vi "Harry_kane_matlab_test.vi"() -> ()   [LabVIEW 2013]
uses:
  <vilib>/imath/engines/lvmath2/RunTimeEngine/ErrorHandling/NIMS_Finalize Error.vi
  <vilib>/imath/engines/lvmath2/RunTimeEngine/Managers/WorkSpace/UID Generator.vi
  <vilib>/imath/engines/lvmath2/RunTimeEngine/VariableToken/NIMS_VariableToken_CondDefined.vi
  <instcachedir>/0/NIMS_VariableToken_CondDefined_9DC5CEC47F8146B087FA2781C705B229.lvgen/NIMS_VariableToken_CondDefined_9DC5CEC47F8146B087FA2781C705B229_001.vi
  <vilib>/imath/engines/lvmath/Functions/Error Handling/MergeErrorsWrapper.vi
  <vilib>/imath/engines/lvmath2/RunTimeEngine/Managers/SymbolTable/Clear UID.vi
  <vilib>/imath/engines/lvmath2/RunTimeEngine/NodeEndStatement/NIMS_NodeEndStatement_Output.vi
  <instcachedir>/0/NIMS_NodeEndStatement_Output_53EC0D466D134D7ABD903AC30B43404B.lvgen/NIMS_NodeEndStatement_Output_53EC0D466D134D7ABD903AC30B43404B_011.vi
  <instcachedir>/0/NIMS_NodeEndStatement_Output_53EC0D466D134D7ABD903AC30B43404B.lvgen/NIMS_NodeEndStatement_Output_53EC0D466D134D7ABD903AC30B43404B_002.vi
  <vilib>/imath/engines/lvmath2/RunTimeEngine/RunTimeType/NIMS_RunTimeType_From StrictType (excl LVString).vi
  <instcachedir>/0/NIMS_RunTimeType_From StrictType (excl LVString)_4DEE718D6EB74582AA20236969C084FC.lvgen/NIMS_RunTimeType_From StrictType (excl LVString)_4DEE718D6EB74582AA20236969C084FC_000.vi
  <vilib>/imath/engines/lvmath2/RunTimeEngine/LocalVariableDefStatement/MC_LocalVariableDefStatement_Display.vi
  <vilib>/imath/engines/lvmath2/RunTimeEngine/IndexRead/NIMS V(S).vi
  <instcachedir>/0/NIMS V(S)_0488751826AF41519A22953C041130DC.lvgen/NIMS V(S)_0488751826AF41519A22953C041130DC_002.vi
  <vilib>/imath/engines/lvmath2/RunTimeEngine/BuiltInFunctions/max/2 inputs/NIMS_max(RG,RG)-no size check.vi
  <instcachedir>/0/NIMS_max(RG,RG)-no size check_F871939977644B7683C1350DCCAD7557.lvgen/NIMS_max(RG,RG)-no size check_F871939977644B7683C1350DCCAD7557_001.vi
  <vilib>/imath/engines/lvmath2/RunTimeEngine/ErrorHandling/NIMS_Create Error From Enums.vi
  <vilib>/imath/engines/lvmath2/RunTimeEngine/RangeToken/NIMS_Range_R2 - Integer.vi
  <instcachedir>/0/NIMS_Range_R2 - Integer_C51C130E5EA5464EA148B28CDAB9615A.lvgen/NIMS_Range_R2 - Integer_C51C130E5EA5464EA148B28CDAB9615A_000.vi
  <vilib>/imath/engines/lvmath2/RunTimeEngine/CommandStatement/MC_CommandStatement_break.vi
  <vilib>/imath/engines/lvmath2/RunTimeEngine/VariableToken/NIMS_VariableToken_CondDefinedDefinedByReplace.vi
  <instcachedir>/0/NIMS_VariableToken_CondDefinedDefinedByReplace_D162CFFC24174562A9FEA619A91E1A56.lvgen/NIMS_VariableToken_CondDefinedDefinedByReplace_D162CFFC24174562A9FEA619A91E1A56_002.vi
  <vilib>/imath/engines/lvmath2/RunTimeEngine/IndexRead/NIMS M(S).vi
  <instcachedir>/0/NIMS M(S)_B826C018497E4940AE96BD27B540B6FB.lvgen/NIMS M(S)_B826C018497E4940AE96BD27B540B6FB_000.vi
  <vilib>/imath/engines/lvmath2/RunTimeEngine/IndexReplace/NIMS V(S)=S.vi
  <instcachedir>/0/NIMS V(S)=S_66A18068148B4981A312229A93EA5C06.lvgen/NIMS V(S)=S_66A18068148B4981A312229A93EA5C06_000.vi
  <instcachedir>/0/NIMS V(S)_0488751826AF41519A22953C041130DC.lvgen/NIMS V(S)_0488751826AF41519A22953C041130DC_000.vi
  <vilib>/imath/engines/lvmath2/RunTimeEngine/BuiltInFunctions/min/2 inputs/NIMS_min(RG,RG)-no size check.vi
  <instcachedir>/0/NIMS_min(RG,RG)-no size check_7F67BAB91AFC452D9517D2EA1C8F5F88.lvgen/NIMS_min(RG,RG)-no size check_7F67BAB91AFC452D9517D2EA1C8F5F88_001.vi
  <vilib>/imathl/engines/lvmath/Functions/Error Handling/Create Error.vi
  <instcachedir>/0/NIMS_VariableToken_CondDefined_9DC5CEC47F8146B087FA2781C705B229.lvgen/NIMS_VariableToken_CondDefined_9DC5CEC47F8146B087FA2781C705B229_003.vi
  <vilib>/imath/engines/lvmath2/RunTimeEngine/BuiltInFunctions/length/NIMS_length(GV).vi
  <instcachedir>/0/NIMS_length(GV)_08A3D13377FD4E4B96F5795FBF3698FA.lvgen/NIMS_length(GV)_08A3D13377FD4E4B96F5795FBF3698FA_000.vi
  <instcachedir>/0/NIMS_VariableToken_CondDefinedDefinedByReplace_D162CFFC24174562A9FEA619A91E1A56.lvgen/NIMS_VariableToken_CondDefinedDefinedByReplace_D162CFFC24174562A9FEA619A91E1A56_001.vi
  <vilib>/imath/engines/lvmath2/RunTimeEngine/IndexReplace/NIMS M(S,S)=S.vi
  <instcachedir>/0/NIMS M(S,S)=S_EC2A86BD47664E68AE45685B0A86CA9E.lvgen/NIMS M(S,S)=S_EC2A86BD47664E68AE45685B0A86CA9E_000.vi
  <vilib>/imath/engines/lvmath2/RunTimeEngine/BuiltInFunctions/length/NIMS_length(GM).vi
  <instcachedir>/0/NIMS_length(GM)_47CEC356FCE0482D9BA47DC61C99F2C7.lvgen/NIMS_length(GM)_47CEC356FCE0482D9BA47DC61C99F2C7_000.vi
  <vilib>/imath/engines/lvmath2/RunTimeEngine/IndexRead/NIMS M(S,S).vi
  <instcachedir>/0/NIMS M(S,S)_AC51E74150A542F7991B9634C66F3096.lvgen/NIMS M(S,S)_AC51E74150A542F7991B9634C66F3096_000.vi
  <vilib>/vision/NI_Vision_Development_Module.lvlib
  <vilib>/imath/engines/lvmath2/RunTimeEngine/Managers/SymbolTable/NIMS_WorkSpace.lvlib
panel:
  in  "Tab Control":enum32{"DIP", "Histogram", "Raw Image"}(tab)
  out "Calibrated":T1(plugin-control)
  in  "Capture image":bool
  in  "Stop":bool
  in  "Calibrate":bool
  out "Puck Array From Reference (cm)":dbl[][](array[numeric])
  out "Player Array From Reference (cm)":dbl[][](array[numeric])
  out "Binary":T1(plugin-control)
  out "Rebound Shots":T1(plugin-control)
  out "Histogram":T2(graph)
  out "Image in":T1(plugin-control)
  out "Puck position pixels":dbl[][](array[numeric])
  out "Player Position Pixels":dbl[][](array[numeric])
  out "appended array":cluster{"X":sgl, "Y":sgl}[](array[cluster])
  out "R":i32
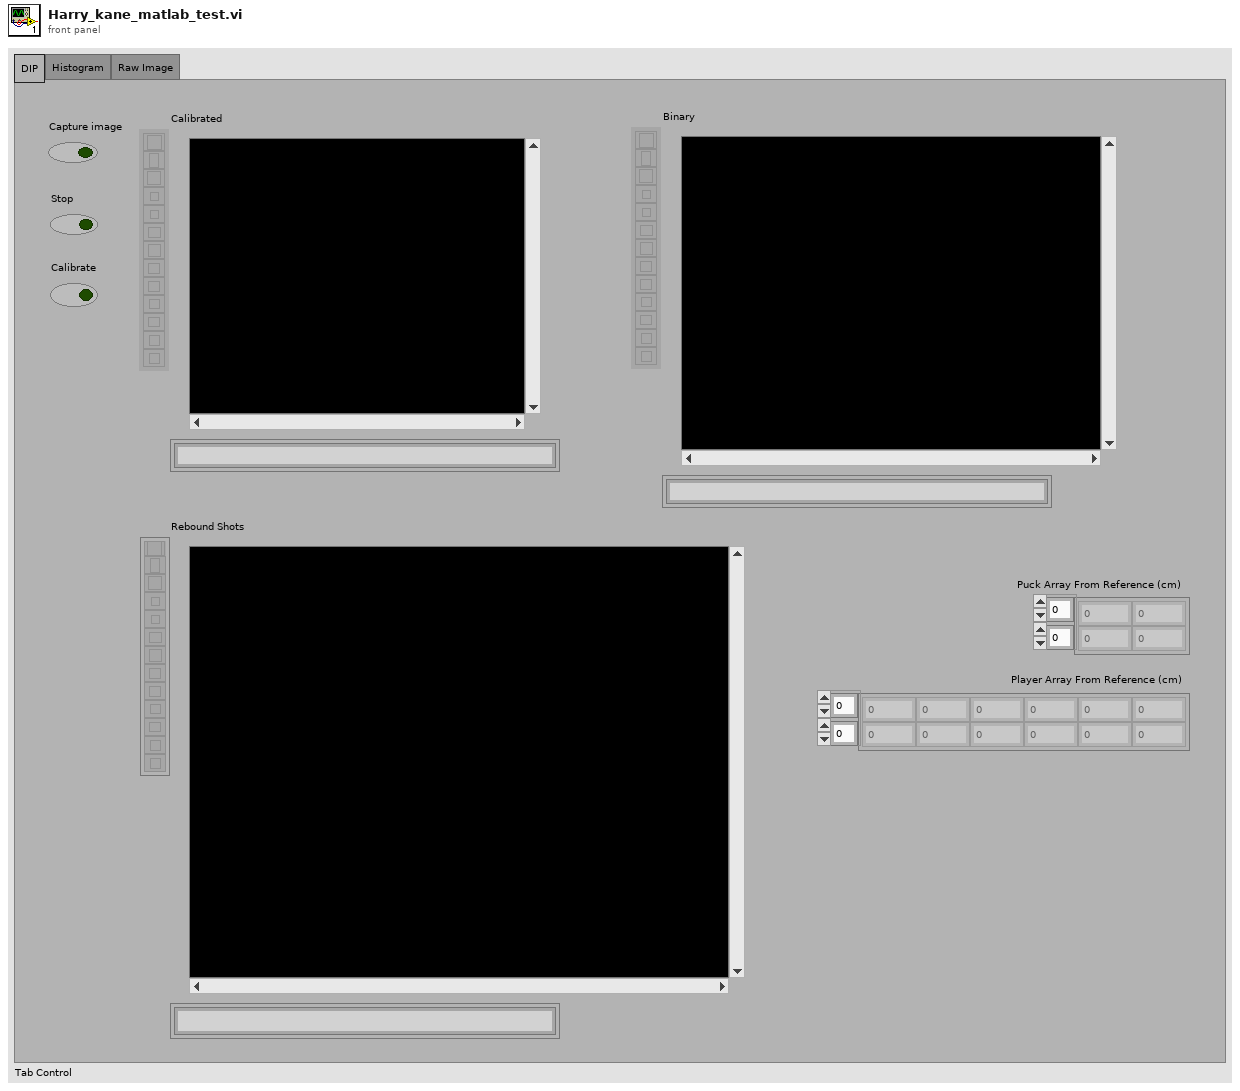
[diagram p1: front panel]
types:
  T1 = typedef "IMAQ Image.ctl" = refnum<image>
  T2 = cluster{"Starting Value":sgl, "Incremental Value":sgl, "Histogram":u32[]}
  T3 = typedef "Image Type" = u32
  T4 = cluster{"Point1 (Pixels)":cluster{"X":sgl, "Y":sgl}, "Point2 (Pixels)":cluster{"X":sgl, "Y":sgl}, "Point1 (Real-World)":cluster{"X":sgl, "Y":sgl}, "Point2 (Real-World)":cluster{"X":sgl, "Y":sgl}, "Angle (Pixel)":dbl, "Angle (Real-World)":dbl, "Score":dbl, "Straightness":dbl, "Average SNR (db)":dbl, "Calibration Valid":bool}
  T5 = cluster{"Start Point":cluster{"X":sgl, "Y":sgl}, "End Point":cluster{"X":sgl, "Y":sgl}, "Length":dbl, "Orientation":dbl, "Score":dbl}[]
  T6 = cluster{"Point1 (Pixels)":cluster{"X":sgl, "Y":sgl}, "Point2 (Pixels)":cluster{"X":sgl, "Y":sgl}}
  T7 = cluster{"Start Point":cluster{"X":sgl, "Y":sgl}, "End Point":cluster{"X":sgl, "Y":sgl}, "Length":dbl, "Orientation":dbl, "Score":dbl}
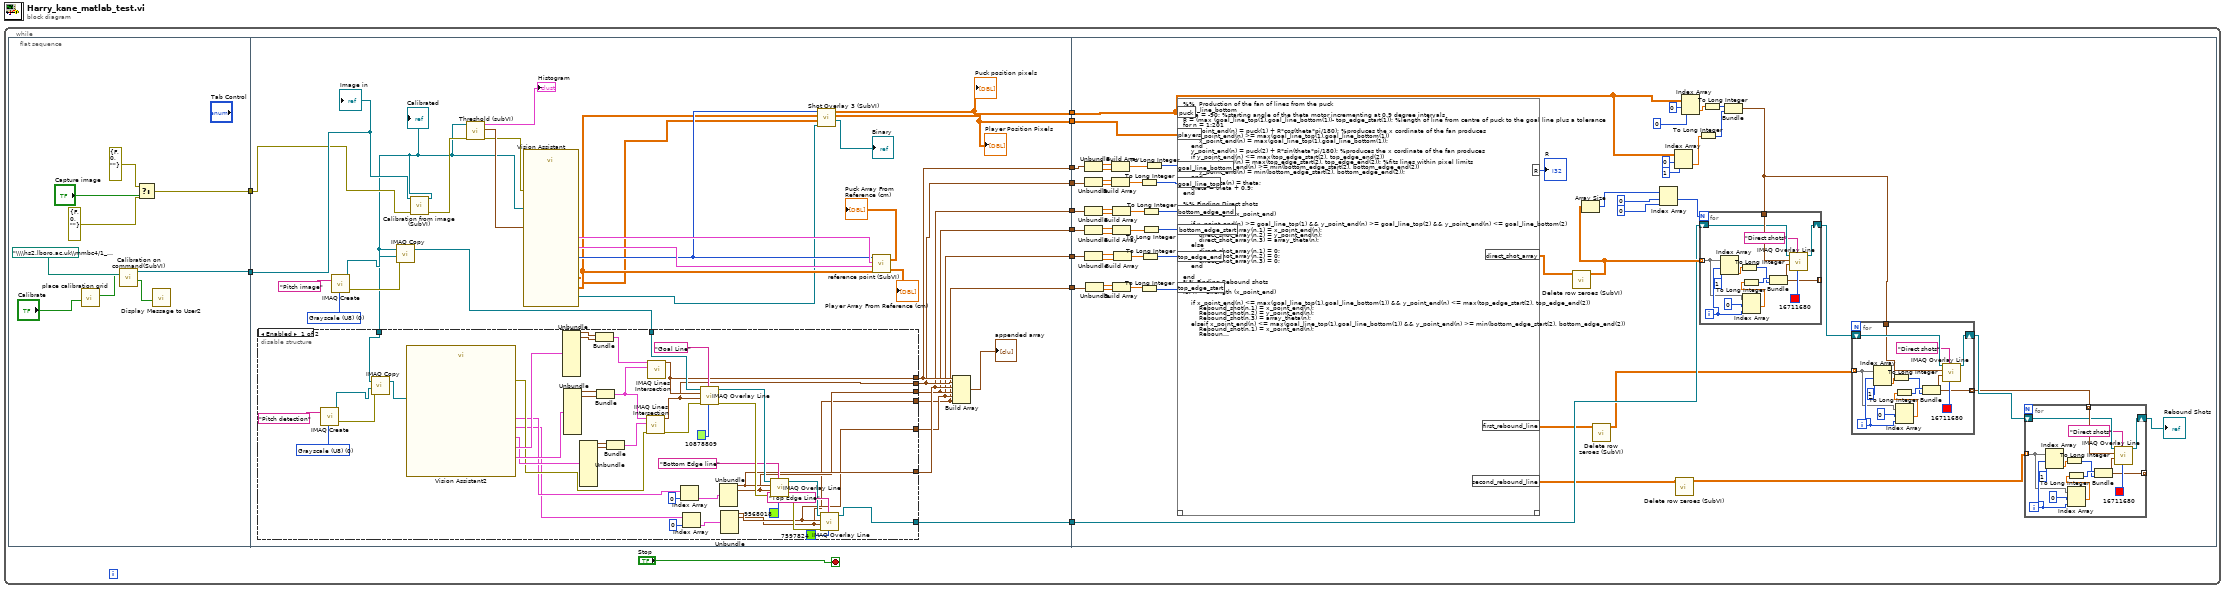
[diagram p0: block diagram]
diagram:
  n1 = while {
    stop <- "Stop" stop-if-true
    n2 = flat-sequence {
      tunnel: [w18] -> w11
      tunnel: [w16] -> w10
      tunnel: w11 -> [w47]
      tunnel: w10 -> [w48]
      tunnel: [w32] -> w9
      tunnel: [w31] -> w8
      tunnel: [w30] -> w7
      tunnel: [w29] -> w6
      tunnel: [w28] -> w5
      tunnel: [w27] -> w4
      tunnel: [w26] -> w3
      tunnel: [w25] -> w2
      tunnel: [w24] -> w1
      tunnel: w9 -> [w120]
      tunnel: w8 -> [w153]
      tunnel: w7 -> [w151]
      tunnel: w6 -> [w148]
      tunnel: w5 -> [w139]
      tunnel: w4 -> [w142]
      tunnel: w3 -> [w141]
      tunnel: w2 -> [w140]
      tunnel: w1 -> [w112]
      frame #0 {
        n3 = call "place calibration grid"("Enable"="Calibrate") -> ("OK"=w14:bool)  [unwired: 9 in, 1 out]
        n4 = call "Calibration on command(SubVI).vi"("Calibrate"=w14, "File Path (Image Calibration 1)"=path "\\\\hs2.lboro.ac.uk\\mmbc4/1_Univesity Work/Mechatronics/Machine Vision/2.0_Harry_kane/Auto_calibration.png") -> ("Boolean"=w13:bool, "Refnum out"=w16:T1)  [unwired: 7 in, 1 out]
        n5 = Select(t=errorcluster {"status"=FALSE, "code"=0, "source"=""} ("error in"), s="Capture image", f=errorcluster {"status"=FALSE, "code"=0, "source"=""} ("error in")) -> (s? t:f=w18:errorcluster)
        n6 = call "Display Message to User2"("Enable"=w13) -> ()  [unwired: 9 in, 2 out]
      }
      frame #1 {
        w37 = T3 0 items=["Grayscale (U8)", "Grayscale (I16)", "Grayscale (SGL)", "Complex (CSG)", "RGB (U32)", "HSL (U32)", "RGB (U64)", "Grayscale (U16)"] ("Image Type")
        n7 = call "IMAQ Create"("Image Name"="Pitch image", "Image Type"=w37) -> ("New Image"=w39:T1, "error out"=w38:errorcluster)  [unwired: 3 in]
        n8 = call "Calibration from image (SubVI).vi"("error in (no error)"=w47, "Refnum in"=w48) -> ("error out"=w46:errorcluster, "Refnum out"=w35:T1)  [unwired: 8 in]
        "Calibrated" <- w35
        n9 = call "IMAQ Copy"("error in (no error)"=w38, "Image Dst"=w39, "Image Src"=w35) -> ("Image Dst Out"=w34:T1)  [unwired: 3 in, 1 out]
        n10 = disable-structure shown="Enabled" {
          disable-tunnel: w35 -> [w96 _]
          disable-tunnel: w34 -> [w74 _]
          disable-tunnel: [w59 _] -> w30
          disable-tunnel: [w58 _] -> w29
          disable-tunnel: [w57 _] -> w28
          disable-tunnel: [w56 _] -> w27
          disable-tunnel: [w55 _] -> w26
          disable-tunnel: [w54 _] -> w25
          disable-tunnel: [w53 _] -> w24
          frame Enabled {
            w93 = T3 0 items=["Grayscale (U8)", "Grayscale (I16)", "Grayscale (SGL)", "Complex (CSG)", "RGB (U32)", "HSL (U32)", "RGB (U64)", "Grayscale (U16)"] ("Image Type")
            n11 = call "IMAQ Create"("Image Name"="Pitch detection", "Image Type"=w93) -> ("New Image"=w95:T1, "error out"=w94:errorcluster)  [unwired: 3 in]
            n12 = call "IMAQ Copy"("error in (no error)"=w94, "Image Dst"=w95, "Image Src"=w96) -> ("Image Dst Out"=w79:T1)  [unwired: 3 in, 1 out]
            n13 = call "Vision Assistant2"("Image In"=w79) -> ("Straight Edge (Top goal edge)"=w83:T4, "Lines (Bottom Edge Detection)"=w73:T5, "Lines (Top Edge Detection)"=w66:T5, "Straight Edge (Bottom goal edge)"=w91:T4, "Straight Edge (Goal Line)"=w87:T4, "error out"=w78:errorcluster)  [unwired: 20 in, 1 out]
            n14 = Unbundle(w91) -> ("Point1 (Pixels)"=w90:cluster{"X":sgl, "Y":sgl}, "Point2 (Pixels)"=w89:cluster{"X":sgl, "Y":sgl})  [unwired: 8 out]
            n15 = Unbundle(w87) -> ("Point1 (Pixels)"=w86:cluster{"X":sgl, "Y":sgl}, "Point2 (Pixels)"=w85:cluster{"X":sgl, "Y":sgl})  [unwired: 8 out]
            n16 = Unbundle(w83) -> ("Point1 (Pixels)"=w82:cluster{"X":sgl, "Y":sgl}, "Point2 (Pixels)"=w81:cluster{"X":sgl, "Y":sgl})  [unwired: 8 out]
            n17 = Bundle("Point1 (Pixels)"=w90, "Point2 (Pixels)"=w89) -> (w88:T6)  [unwired: 1 in]
            n18 = Bundle("Point1 (Pixels)"=w86, "Point2 (Pixels)"=w85) -> (w84:T6)  [unwired: 1 in]
            n19 = Bundle("Point1 (Pixels)"=w82, "Point2 (Pixels)"=w81) -> (w80:T6)  [unwired: 1 in]
            n20 = call "IMAQ Lines Intersection"("error in (no error)"=w78, "Line 2"=w80, "Line 1"=w84) -> ("error out"=w77:errorcluster, "Intersection Point"=w58:cluster{"X":sgl, "Y":sgl})  [unwired: 6 in, 1 out]
            n21 = call "IMAQ Lines Intersection"("Line 2"=w84, "Line 1"=w88) -> ("Intersection Point"=w59:cluster{"X":sgl, "Y":sgl})  [unwired: 7 in, 2 out]
            n22 = Index Array(array=w73, index=0) -> (element=w71:T7)
            n23 = Index Array(array=w66, index=0) -> (element=w64:T7)
            n24 = call "IMAQ Overlay Line"("Color"=u32 10878809, "Group"="Goal Line", "error in (no error)"=w77, "End Point"=w58, "Start Point"=w59, "Image"=w74) -> ("error out"=w70:errorcluster, "Image Out"=w69:T1)  [unwired: 4 in]
            n25 = Unbundle(w71) -> ("Start Point"=w57:cluster{"X":sgl, "Y":sgl}, "End Point"=w56:cluster{"X":sgl, "Y":sgl})  [unwired: 3 out]
            n26 = Unbundle(w64) -> ("Start Point"=w55:cluster{"X":sgl, "Y":sgl}, "End Point"=w54:cluster{"X":sgl, "Y":sgl})  [unwired: 3 out]
            n27 = call "IMAQ Overlay Line"("Color"=u32 9568018, "Group"="Bottom Edge line", "error in (no error)"=w70, "End Point"=w56, "Start Point"=w57, "Image"=w69) -> ("error out"=w63:errorcluster, "Image Out"=w60:T1)  [unwired: 4 in]
            n28 = call "IMAQ Overlay Line"("Color"=u32 7597824, "Group"="Top Edge Line", "error in (no error)"=w63, "End Point"=w54, "Start Point"=w55, "Image"=w60) -> ("Image Out"=w53:T1)  [unwired: 4 in, 1 out]
          }
          frame Disabled {
          }
        }
        n29 = call "Threshold (subVI).vi"("error in (no error)"=w46, "Image  in"=w35) -> ("error out"=w45:errorcluster, "Cluster"=w52:cluster{sgl, "element":sgl}, "Histogram"=→"Histogram":T2)  [unwired: 7 in]
        n30 = call "Vision Assistant"("Image In"=w35, "Range (Threshold 1)"=w52, "error in"=w45) -> ("Image Out"=w23:T1, "Particle Measurements (Real-World) (Particle Analysis 1)"=w41:dbl[][], "Particle Measurements (Pixels) (Particle Analysis 1)"=w40:dbl[][], "Straight Edge (Find Straight Edge 1)"=w50:T4, "Straight Edge (Find Straight Edge 2)"=w49:T4, "Nb Circles (Circle Detection 1)"=w42:i32)  [unwired: 17 in, 2 out]
        n31 = call "Shot Overlay 3 (SubVI).vi"("Image Out"=w23, "Particle Measurements (Pixels) (Particle Analysis 1)"=w40, "Particle Measurements (Real-World) (Particle Analysis 1)"=w41, "Nb Circles (Circle Detection 1)"=w42) -> ("Player area overlay"=→"Binary":T1, "Player Position Pixels"=w31:dbl[][], "Puck position pixels"=w32:dbl[][])  [unwired: 3 in]
        "Puck position pixels" <- w32
        "Player Position Pixels" <- w31
        n32 = call "reference point (SubVI).vi"("Nb Circles (Circle Detection 1)"=w42, "Straight Edge (Find Straight Edge 1)"=w50, "Straight Edge (Find Straight Edge 2)"=w49, "Particle Measurements (Real-World) (Particle Analysis 1)"=w41) -> ("Puck X, Y co-ordinates"=→"Puck Array From Reference (cm)":dbl[][], "Player X, Y co-ordinates"=→"Player Array From Reference (cm)":dbl[][])  [unwired: 1 in]
        n33 = Build Array(w30, w29, w28, w27, w26, w25) -> (→"appended array":cluster{"X":sgl, "Y":sgl}[])
        "Image in" <- w48
      }
      frame #2 {
        n34 = Unbundle(w139) -> ("X"=w138:sgl, "Y"=w137:sgl)
        n35 = Unbundle(w141) -> ("X"=w133:sgl, "Y"=w128:sgl)
        n36 = Unbundle(w151) -> ("X"=w150:sgl, "Y"=w149:sgl)
        n37 = Unbundle(w148) -> ("X"=w147:sgl, "Y"=w146:sgl)
        n38 = Unbundle(w142) -> ("X"=w134:sgl, "Y"=w125:sgl)
        n39 = Unbundle(w140) -> ("X"=w132:sgl, "Y"=w131:sgl)
        n40 = Build Array(w150, w149) -> (w144:sgl[])
        n41 = Build Array(w147, w146) -> (w145:sgl[])
        n42 = Build Array(w138, w137) -> (w136:sgl[])
        n43 = Build Array(w134, w125) -> (w124:sgl[])
        n44 = Build Array(w132, w131) -> (w130:sgl[])
        n45 = Build Array(w133, w128) -> (w127:sgl[])
        n46 = To Long Integer(number=w145) -> (32bit integer=w152:i32[])
        n47 = To Long Integer(number=w130) -> (32bit integer=w129:i32[])
        n48 = To Long Integer(number=w127) -> (32bit integer=w126:i32[])
        n49 = To Long Integer(number=w124) -> (32bit integer=w123:i32[])
        n50 = To Long Integer(number=w136) -> (32bit integer=w135:i32[])
        n51 = To Long Integer(number=w144) -> (32bit integer=w143:i32[])
        n52 = mathscript code="%%  Production of the fan of lines from the puck \ngoal_line_bottom\ntheta = -90; %starting angle of the theta motor incrementing at 0.9 degree intervals\nR = (max (goal_line_top(1),goal_line_bottom(1))- top_edge_start(1)); %length of line from centre of puck to the goal line plus a tolerance\nfor n = 1:201\n    x_point_end(n) = puck(1) + R*cos(theta*pi/180); %produces the x cordinate of the fan produces\n    if x_point_end(n) >= max(goal_line_top(1),goal_line_bottom(1))\n        x_point_end(n) = max(goal_line_top(1),goal_line_bottom(1));\n    end\n    y_point_end(n) = puck(2) + R*sin(theta*pi/180); %produces the x cordinate of the fan produces\n    if y_point_end(n) <= max(top_edge_start(2), top_edge_end(2))\n       y_point_end(n) = max(top_edge_start(2), top_edge_end(2)); %fits lines within pixel limits\n    elseif y_point_end(n) >= min(bottom_edge_start(2), bottom_edge_end(2))\n        y_point_end(n) = min(bottom_edge_start(2), bottom_edge_end(2));\n    end \n    array_theta(n) = theta;\n    theta = theta + 0.9;\nend\n\n%% Finding Direct shots\n\nfor n = 1:length (x_point_end)\n   \n    if x_point_end(n) >= goal_line_top(1) && y_point_end(n) >= goal_line_top(2) && y_point_end(n) <= goal_line_bottom(2)\n        direct_shot_array(n,1) = x_point_end(n);\n        direct_shot_array(n,2) = y_point_end(n);\n        direct_shot_array(n,3) = array_theta(n);\n    else\n        direct_shot_array(n,1) = 0;\n        direct_shot_array(n,2) = 0;\n        direct_shot_array(n,3) = 0;\n    end\n    \nend\n%% Finding Rebound shots \n\nfor n = 1:length (x_point_end)\n   \n    if x_point_end(n) <= max(goal_line_top(1),goal_line_bottom(1)) && y_point_end(n) <= max(top_edge_start(2), top_edge_end(2))\n        Rebound_shot(n,1) = x_point_end(n);\n        Rebound_shot(n,2) = y_point_end(n);\n        Rebound_shot(n,3) = array_theta(n);\n    elseif x_point_end(n) <= max(goal_line_top(1),goal_line_bottom(1)) && y_point_end(n) >= min(bottom_edge_start(2), bottom_edge_end(2))\n        Rebound_shot(n,1) = x_point_end(n);\n        Rebound_shot(n,2) = y_point_end(n);\n        Rebound_shot(n,3) = array_theta(n);\n    else\n        Rebound_shot(n,1) = 0;\n        Rebound_shot(n,2) = 0;\n        Rebound_shot(n,3) = 0;\n    end    \nend\n%Rebound_shot( any(Rebound_shot,2), : ) = [];  %rows\n\n%% Calculating rebound trajectory\nR_rebound = bottom_edge_start(2) - top_edge_start(2);\n\nfor n = 1:length(Rebound_shot)\n\n     x = max(goal_line_top(1),goal_line_bottom(1)) - Rebound_shot(n,1);\n    Rebound_y_end(n) =  Rebound_shot(n,2) + x*(tan(-1*Rebound_shot(n,3)*pi/180));\n    \n    if  Rebound_y_end(n) >= goal_line_top(2) && Rebound_y_end(n) <= goal_line_bottom(2)\n        first_rebound_line(n,1) = Rebound_shot(n,1);\n        first_rebound_line(n,2) = Rebound_shot(n,2);\n        first_rebound_line(n,3) = Rebound_shot(n,3);\n        second_rebound_line(n,1) = max(goal_line_top(1),goal_line_bottom(1));\n        second_rebound_line(n,2) = Rebound_y_end(n);\n    else\n        first_rebound_line(n,1) = 0;\n        first_rebound_line(n,2) = 0;\n        first_rebound_line(n,3) = 0;\n        second_rebound_line(n,1) = 0;\n        second_rebound_line(n,2) = 0;\n    end\n   \n \nend"("puck"=w120, "players"=w153, "goal_line_top"=w152, "goal_line_bottom"=w143, "bottom_edge_end"=w135, "bottom_edge_start"=w123, "top_edge_end"=w126, "top_edge_start"=w129) -> ("direct_shot_array"=w107:dbl[][], "first_rebound_line"=w106:dbl[][], "second_rebound_line"=w102:dbl[][], "R"=→"R":i32)  [unwired: 1 in, 1 out]
        n53 = call "Delete row zeroes (SubVI).vi"("direct_shot_array"=w107) -> ("Array"=w117:dbl[][])  [unwired: 10 in]
        n54 = Array Size(array=w117) -> (size(s)=w116:i32[])
        n55 = call "Delete row zeroes (SubVI).vi"("direct_shot_array"=w106) -> ("Array"=w105:dbl[][])  [unwired: 10 in]
        n56 = Index Array(array=w116, index #1=0 ("index"), index #2=0 ("index")) -> (element #1=w114:i32)  [unwired: 1 out]
        n57 = Index Array(array=w120, index (row)=0, index (col)=1 ("disabled index (col)")) -> (element=w109:dbl)
        n58 = call "Delete row zeroes (SubVI).vi"("direct_shot_array"=w102) -> ("Array"=w99:dbl[][])  [unwired: 10 in]
        n59 = Index Array(array=w120, index (row)=0, index (col)=0 ("disabled index (col)")) -> (element=w111:dbl)
        n60 = To Long Integer(number=w109) -> (32bit integer=w108:i32)
        n61 = To Long Integer(number=w111) -> (32bit integer=w110:i32)
        n62 = Bundle(w110, w108) -> (w100:cluster{i32, i32})  [unwired: 1 in]
        n63 = for {
          N: w114 -> [_]
          tunnel: w117 -> [w190] mode=indexing
          tunnel: w100 -> [w195]
          shift-right: [w189] -> w104
          shift-left: w112 -> [w194]
          tunnel: [w186] -> _ mode=indexing
          i -> [w191]
          n64 = Index Array(array=w190, index #1=w191, index #2=1 ("index")) -> (element #2=w182:dbl)  [unwired: 1 out]
          n65 = To Long Integer(number=w182) -> (32bit integer=w183:i32)
          n66 = Index Array(array=w190, index #1=0 ("index"), index #2=w191) -> (element #1=w185:dbl)  [unwired: 1 out]
          n67 = To Long Integer(number=w185) -> (32bit integer=w184:i32)
          n68 = Bundle(w184, w183) -> (w186:cluster{i32, i32})  [unwired: 1 in]
          n69 = call "IMAQ Overlay Line"("Color"=u32 16711680, "Group"="Direct shots", "End Point"=w186, "Start Point"=w195, "Image"=w194) -> ("Image Out"=w189:T1)  [unwired: 5 in, 1 out]
        }
        n70 = for {
          tunnel: w105 -> [w177] mode=indexing
          shift-right: [w176] -> w101
          shift-left: w104 -> [w181]
          tunnel: [w173] -> w97 mode=indexing
          tunnel: w100 -> [w168]
          i -> [w178]
          n71 = Index Array(array=w177, index #1=w178, index #2=1 ("index")) -> (element #2=w169:dbl)  [unwired: 1 out]
          n72 = To Long Integer(number=w169) -> (32bit integer=w170:i32)
          n73 = Index Array(array=w177, index #1=0 ("index"), index #2=w178) -> (element #1=w172:dbl)  [unwired: 1 out]
          n74 = To Long Integer(number=w172) -> (32bit integer=w171:i32)
          n75 = Bundle(w171, w170) -> (w173:cluster{i32, i32})  [unwired: 1 in]
          n76 = call "IMAQ Overlay Line"("Color"=u32 16711680, "Group"="Direct shots", "End Point"=w173, "Start Point"=w168, "Image"=w181) -> ("Image Out"=w176:T1)  [unwired: 5 in, 1 out]
        }
        n77 = for {
          tunnel: w99 -> [w162] mode=indexing
          tunnel: w97 -> [w167] mode=indexing
          shift-right: [w161] -> w98
          shift-left: w101 -> [w166]
          tunnel: [w158] -> _ mode=indexing
          i -> [w163]
          n78 = Index Array(array=w162, index #1=w163, index #2=1 ("index")) -> (element #2=w154:dbl)  [unwired: 1 out]
          n79 = To Long Integer(number=w154) -> (32bit integer=w155:i32)
          n80 = Index Array(array=w162, index #1=0 ("index"), index #2=w163) -> (element #1=w157:dbl)  [unwired: 1 out]
          n81 = To Long Integer(number=w157) -> (32bit integer=w156:i32)
          n82 = Bundle(w156, w155) -> (w158:cluster{i32, i32})  [unwired: 1 in]
          n83 = call "IMAQ Overlay Line"("Color"=u32 16711680, "Group"="Direct shots", "End Point"=w158, "Start Point"=w167, "Image"=w166) -> ("Image Out"=w161:T1)  [unwired: 5 in, 1 out]
        }
        "Rebound Shots" <- w98
      }
    }
  }
